vi "Load Layout By Name.vi"(8 "error in (no error)":errorcluster, 10 "key":string, 11 "Cluster":T6) -> (0 "error out":errorcluster)   [LabVIEW 2020, in "MDI ViewManager.lvlib"]
uses:
  MDI ViewManager.lvlib
  Typedef/Layout.ctl
  <vilib>/Utility/miscctls.llb/LVPointTypeDef.ctl
  <vilib>/Utility/miscctls.llb/LVBoundsTypeDef.ctl
  <vilib>/Utility/miscctls.llb/LVPositionTypeDef.ctl
  Typedef/Update View.ctl
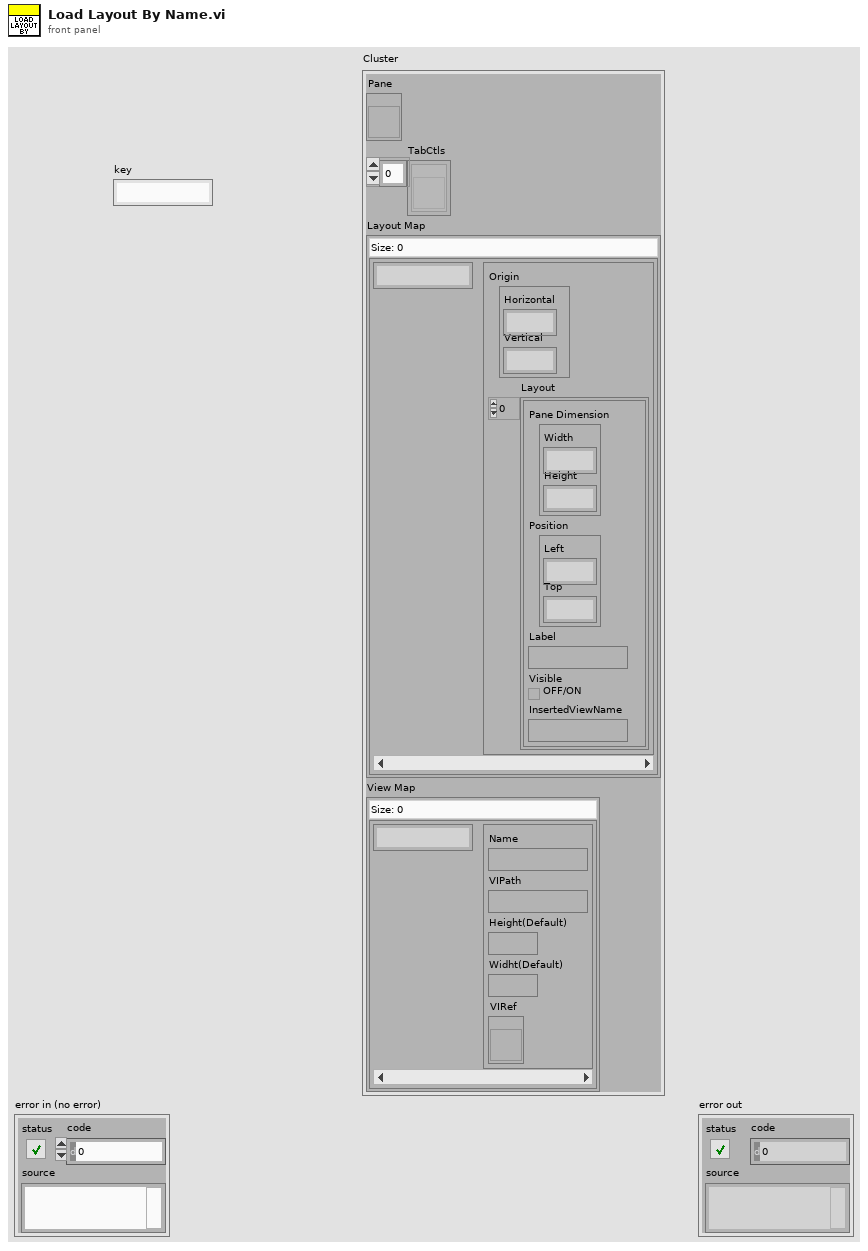
[diagram p1: front panel]
types:
  T1 = typedef "MDI ViewManager.lvlib/Layout.ctl" = cluster{"Origin":T2, "Layout":cluster{"Pane Dimension":T3, "Position":T4, "Label":string, "Visible":bool, "InsertedViewName":string}[]}
  T2 = typedef "LVPointTypeDef.ctl" = cluster{"Horizontal":i16, "Vertical":i16}
  T3 = typedef "LVBoundsTypeDef.ctl" = cluster{"Width":u32, "Height":u32}
  T4 = typedef "LVPositionTypeDef.ctl" = cluster{"Left":i32, "Top":i32}
  T5 = typedef "MDI ViewManager.lvlib/Update View.ctl" = cluster{"Name":string, "VIPath":path, "Height(Default)":u32, "Widht(Default)":u32, "VIRef":refnum<vi>}
  T6 = cluster{"Pane":refnum<vi>, "TabCtls":refnum<vi>[], "Layout Map":map{string, T1}, "View Map":map{string, T5}}
  T7 = cluster{"Pane Dimension":T3, "Position":T4, "Label":string, "Visible":bool, "InsertedViewName":string}[]
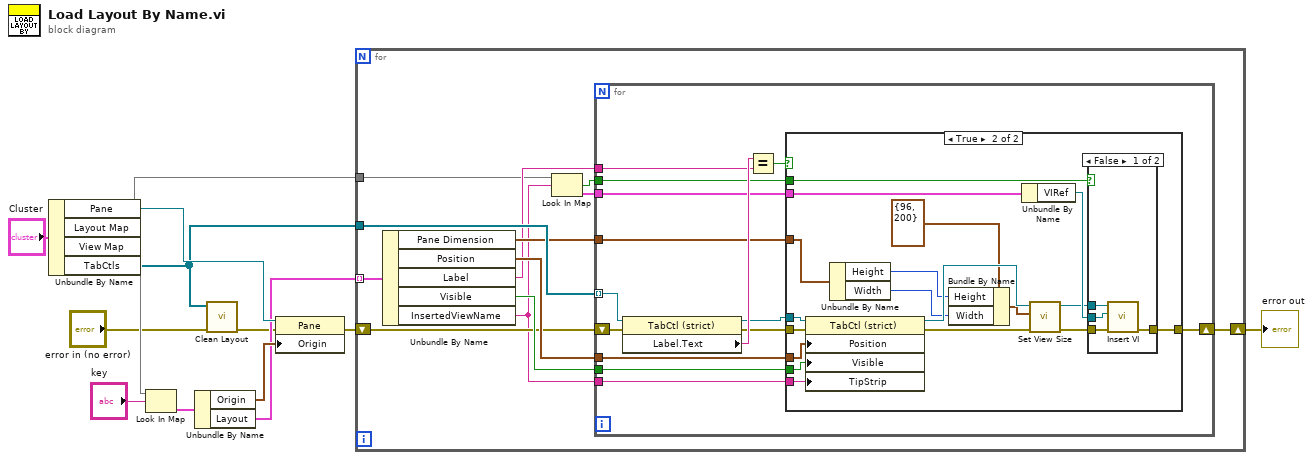
[diagram p0: block diagram]
diagram:
  n1 = Unbundle By Name("Cluster") -> ("Pane"=w12:refnum<vi>, "Layout Map"=w11:map{string, T1}, "View Map"=w6:map{string, T5}, "TabCtls"=w1:refnum<vi>[])
  n2 = Look In Map(map=w11, key="key") -> (value=w9:T1)  [unwired: 1 in, 1 out]
  n3 = Unbundle By Name(w9) -> ("Origin"=w8:T2, "Layout"=w7:T7)
  n4 = call "Clean Layout.vi"("error in (no error)"="error in (no error)", "TabCtls"=w1) -> ("error out"=w2:errorcluster)  [unwired: 9 in]
  n5 = property class="Pane"(reference=w12, error in=w2, "Origin"=w8) -> (error out=w5:errorcluster)  [unwired: 1 out]
  n6 = for {
    tunnel: w7 -> [w24] mode=indexing
    tunnel: w1 -> [w25]
    tunnel: w6 -> [w17]
    shift-right: [w18] -> w4
    shift-left: w5 -> [w19]
    n7 = Unbundle By Name(w24) -> ("Pane Dimension"=w23:T3, "Position"=w22:T4, "Label"=w20:string, "Visible"=w21:bool, "InsertedViewName"=w16:string)
    n8 = Look In Map(map=w17, key=w16) -> (key not found?=w14:bool, value=w15:T5)  [unwired: 1 in]
    n9 = for {
      tunnel: w25 -> [w39] mode=indexing
      tunnel: w23 -> [w36]
      tunnel: w22 -> [w35]
      tunnel: w20 -> [w34]
      tunnel: w21 -> [w33]
      tunnel: w16 -> [w32]
      tunnel: w15 -> [w31]
      shift-right: [w30] -> w18
      shift-left: w19 -> [w28]
      tunnel: w14 -> [w26]
      n10 = property class="TabCtl (strict)"(reference=w39, error in=w28) -> (reference out=w29:refnum<vi>, error out=w27:errorcluster, "Label.Text"=w38:string)
      n11 = Equal?(x=w38, y=w34) -> (x = y?=w37:bool)
      n12 = case shown="True" w37 {
        tunnel: w36 -> [_ w55]
        tunnel: w35 -> [_ w58]
        tunnel: w33 -> [_ w57]
        tunnel: w29 -> [_ w56]
        tunnel: w32 -> [_ w53]
        tunnel: w31 -> [_ w52]
        tunnel: w27 -> [w40 w51]
        tunnel: [w40 w50] -> w30
        tunnel: w26 -> [_ w49]
        frame False {
        }
        frame True {
          n13 = property class="TabCtl (strict)"(reference=w56, error in=w51, "Position"=w58, "Visible"=w57, "TipStrip"=w53) -> (reference out=w48:refnum<vi>, error out=w45:errorcluster)
          n14 = Unbundle By Name(w55) -> ("Height"=w42:u32, "Width"=w41:u32)
          n15 = Bundle By Name(cluster=T3 {"Width"=96, "Height"=200} ("TabDimension"), "Height"=w42, "Width"=w41) -> (w43:T3)
          n16 = Unbundle By Name(w52) -> ("VIRef"=w54:refnum<vi>)
          n17 = call "Set View Size.vi"("error in (no error)"=w45, "TabDimension"=w43, "TabControlRef in"=w48) -> ("error out"=w46:errorcluster, "TabControlRef out"=w47:refnum<vi>)  [unwired: 7 in]
          n18 = case shown="False" w49 {
            tunnel: w54 -> [w62 _]
            tunnel: w47 -> [w61 _]
            tunnel: w46 -> [w60 w63]
            tunnel: [w59 w63] -> w50
            frame False {
              n19 = call "Insert VI.vi"("error in (no error)"=w60, "VIRef"=w62, "TabControl in"=w61) -> ("error out"=w59:errorcluster)  [unwired: 7 in, 1 out]
            }
            frame True {
            }
          }
        }
      }
    }
  }
  "error out" <- w4
